vi "DAQ_software.vi"() -> ()   [LabVIEW 2014]
uses:
  <vilib>/Utility/file.llb/Write To Spreadsheet File (string).vi
panel:
  in  "recTime":dbl
  out "elapsed time":string
  out "end time":string
  out "start time":string
  out "Plot 6":waveform(dbl)(graph)={"t0"=timestamp(3541407835.153924 s since 1904-01-01), "dt"=0.001, "Y"=[-0.04272921159212641, -0.04272921159212641, -0.04305886997433487, -0.04305886997433487, -0.04305886997433487, -0.0433885283565454, -0.04305886997433487, -0.04305886997433487, -0.043718186738758026, -0.0433885283565454, -0.04305886997433487, -0.04239955320992001, -0.04239955320992001, -0.04239955320992001, -0.04305886997433487, -0.04272921159212641, -0.04239955320992001, -0.04272921159212641, -0.04206989482771564, -0.04272921159212641, -0.04272921159212641, -0.04272921159212641, -0.04272921159212641, -0.04272921159212641, -0.04272921159212641, -0.04239955320992001, -0.04272921159212641, -0.04272921159212641, -0.04272921159212641, -0.04272921159212641, -0.04305886997433487, -0.04305886997433487, -0.04305886997433487, -0.04272921159212641, -0.04272921159212641, -0.04305886997433487, -0.04272921159212641, -0.04305886997433487, -0.04272921159212641, -0.04239955320992001, -0.04272921159212641, -0.04305886997433487, -0.04272921159212641, -0.04272921159212641, -0.04305886997433487, -0.04305886997433487, -0.04272921159212641, -0.04206989482771564, -0.04272921159212641, -0.04305886997433487, -0.04272921159212641, -0.04239955320992001, -0.04239955320992001, -0.04272921159212641, -0.04272921159212641, -0.04239955320992001, -0.04239955320992001, -0.04272921159212641, -0.04239955320992001, -0.04272921159212641, -0.04239955320992001, -0.04272921159212641, -0.04239955320992001, -0.04239955320992001, -0.04239955320992001, -0.04305886997433487, -0.04305886997433487, -0.04305886997433487, -0.04305886997433487, -0.04272921159212641, -0.04305886997433487, -0.04272921159212641, -0.04239955320992001, -0.04239955320992001, -0.04305886997433487, -0.04239955320992001, -0.04239955320992001, -0.04239955320992001, -0.04239955320992001, -0.04272921159212641, -0.04272921159212641, -0.04239955320992001, -0.04239955320992001, -0.04239955320992001, -0.04239955320992001, -0.04239955320992001, -0.04239955320992001, -0.04272921159212641, -0.04272921159212641, -0.04305886997433487, -0.04272921159212641, -0.04272921159212641, -0.04272921159212641, -0.04272921159212641, -0.04272921159212641, -0.04272921159212641, -0.04239955320992001, -0.04239955320992001, -0.04272921159212641, -0.04272921159212641], "attributes"=variant("NI_ChannelName"=variant(string "ch1"), "NI_UnitDescription"=variant(string "Volts"))}
  out "Plot 5":waveform(dbl)(graph)={"t0"=timestamp(3541407835.153924 s since 1904-01-01), "dt"=0.001, "Y"=[-0.04272921159212641, -0.04272921159212641, -0.04305886997433487, -0.04305886997433487, -0.04305886997433487, -0.0433885283565454, -0.04305886997433487, -0.04305886997433487, -0.043718186738758026, -0.0433885283565454, -0.04305886997433487, -0.04239955320992001, -0.04239955320992001, -0.04239955320992001, -0.04305886997433487, -0.04272921159212641, -0.04239955320992001, -0.04272921159212641, -0.04206989482771564, -0.04272921159212641, -0.04272921159212641, -0.04272921159212641, -0.04272921159212641, -0.04272921159212641, -0.04272921159212641, -0.04239955320992001, -0.04272921159212641, -0.04272921159212641, -0.04272921159212641, -0.04272921159212641, -0.04305886997433487, -0.04305886997433487, -0.04305886997433487, -0.04272921159212641, -0.04272921159212641, -0.04305886997433487, -0.04272921159212641, -0.04305886997433487, -0.04272921159212641, -0.04239955320992001, -0.04272921159212641, -0.04305886997433487, -0.04272921159212641, -0.04272921159212641, -0.04305886997433487, -0.04305886997433487, -0.04272921159212641, -0.04206989482771564, -0.04272921159212641, -0.04305886997433487, -0.04272921159212641, -0.04239955320992001, -0.04239955320992001, -0.04272921159212641, -0.04272921159212641, -0.04239955320992001, -0.04239955320992001, -0.04272921159212641, -0.04239955320992001, -0.04272921159212641, -0.04239955320992001, -0.04272921159212641, -0.04239955320992001, -0.04239955320992001, -0.04239955320992001, -0.04305886997433487, -0.04305886997433487, -0.04305886997433487, -0.04305886997433487, -0.04272921159212641, -0.04305886997433487, -0.04272921159212641, -0.04239955320992001, -0.04239955320992001, -0.04305886997433487, -0.04239955320992001, -0.04239955320992001, -0.04239955320992001, -0.04239955320992001, -0.04272921159212641, -0.04272921159212641, -0.04239955320992001, -0.04239955320992001, -0.04239955320992001, -0.04239955320992001, -0.04239955320992001, -0.04239955320992001, -0.04272921159212641, -0.04272921159212641, -0.04305886997433487, -0.04272921159212641, -0.04272921159212641, -0.04272921159212641, -0.04272921159212641, -0.04272921159212641, -0.04272921159212641, -0.04239955320992001, -0.04239955320992001, -0.04272921159212641, -0.04272921159212641], "attributes"=variant("NI_ChannelName"=variant(string "ch1"), "NI_UnitDescription"=variant(string "Volts"))}
  out "Plot 4":waveform(dbl)(graph)={"t0"=timestamp(3541407835.153924 s since 1904-01-01), "dt"=0.001, "Y"=[-0.04272921159212641, -0.04272921159212641, -0.04305886997433487, -0.04305886997433487, -0.04305886997433487, -0.0433885283565454, -0.04305886997433487, -0.04305886997433487, -0.043718186738758026, -0.0433885283565454, -0.04305886997433487, -0.04239955320992001, -0.04239955320992001, -0.04239955320992001, -0.04305886997433487, -0.04272921159212641, -0.04239955320992001, -0.04272921159212641, -0.04206989482771564, -0.04272921159212641, -0.04272921159212641, -0.04272921159212641, -0.04272921159212641, -0.04272921159212641, -0.04272921159212641, -0.04239955320992001, -0.04272921159212641, -0.04272921159212641, -0.04272921159212641, -0.04272921159212641, -0.04305886997433487, -0.04305886997433487, -0.04305886997433487, -0.04272921159212641, -0.04272921159212641, -0.04305886997433487, -0.04272921159212641, -0.04305886997433487, -0.04272921159212641, -0.04239955320992001, -0.04272921159212641, -0.04305886997433487, -0.04272921159212641, -0.04272921159212641, -0.04305886997433487, -0.04305886997433487, -0.04272921159212641, -0.04206989482771564, -0.04272921159212641, -0.04305886997433487, -0.04272921159212641, -0.04239955320992001, -0.04239955320992001, -0.04272921159212641, -0.04272921159212641, -0.04239955320992001, -0.04239955320992001, -0.04272921159212641, -0.04239955320992001, -0.04272921159212641, -0.04239955320992001, -0.04272921159212641, -0.04239955320992001, -0.04239955320992001, -0.04239955320992001, -0.04305886997433487, -0.04305886997433487, -0.04305886997433487, -0.04305886997433487, -0.04272921159212641, -0.04305886997433487, -0.04272921159212641, -0.04239955320992001, -0.04239955320992001, -0.04305886997433487, -0.04239955320992001, -0.04239955320992001, -0.04239955320992001, -0.04239955320992001, -0.04272921159212641, -0.04272921159212641, -0.04239955320992001, -0.04239955320992001, -0.04239955320992001, -0.04239955320992001, -0.04239955320992001, -0.04239955320992001, -0.04272921159212641, -0.04272921159212641, -0.04305886997433487, -0.04272921159212641, -0.04272921159212641, -0.04272921159212641, -0.04272921159212641, -0.04272921159212641, -0.04272921159212641, -0.04239955320992001, -0.04239955320992001, -0.04272921159212641, -0.04272921159212641], "attributes"=variant("NI_ChannelName"=variant(string "ch1"), "NI_UnitDescription"=variant(string "Volts"))}
  out "Plot 3":waveform(dbl)(graph)={"t0"=timestamp(3541407835.153924 s since 1904-01-01), "dt"=0.001, "Y"=[-0.04272921159212641, -0.04272921159212641, -0.04305886997433487, -0.04305886997433487, -0.04305886997433487, -0.0433885283565454, -0.04305886997433487, -0.04305886997433487, -0.043718186738758026, -0.0433885283565454, -0.04305886997433487, -0.04239955320992001, -0.04239955320992001, -0.04239955320992001, -0.04305886997433487, -0.04272921159212641, -0.04239955320992001, -0.04272921159212641, -0.04206989482771564, -0.04272921159212641, -0.04272921159212641, -0.04272921159212641, -0.04272921159212641, -0.04272921159212641, -0.04272921159212641, -0.04239955320992001, -0.04272921159212641, -0.04272921159212641, -0.04272921159212641, -0.04272921159212641, -0.04305886997433487, -0.04305886997433487, -0.04305886997433487, -0.04272921159212641, -0.04272921159212641, -0.04305886997433487, -0.04272921159212641, -0.04305886997433487, -0.04272921159212641, -0.04239955320992001, -0.04272921159212641, -0.04305886997433487, -0.04272921159212641, -0.04272921159212641, -0.04305886997433487, -0.04305886997433487, -0.04272921159212641, -0.04206989482771564, -0.04272921159212641, -0.04305886997433487, -0.04272921159212641, -0.04239955320992001, -0.04239955320992001, -0.04272921159212641, -0.04272921159212641, -0.04239955320992001, -0.04239955320992001, -0.04272921159212641, -0.04239955320992001, -0.04272921159212641, -0.04239955320992001, -0.04272921159212641, -0.04239955320992001, -0.04239955320992001, -0.04239955320992001, -0.04305886997433487, -0.04305886997433487, -0.04305886997433487, -0.04305886997433487, -0.04272921159212641, -0.04305886997433487, -0.04272921159212641, -0.04239955320992001, -0.04239955320992001, -0.04305886997433487, -0.04239955320992001, -0.04239955320992001, -0.04239955320992001, -0.04239955320992001, -0.04272921159212641, -0.04272921159212641, -0.04239955320992001, -0.04239955320992001, -0.04239955320992001, -0.04239955320992001, -0.04239955320992001, -0.04239955320992001, -0.04272921159212641, -0.04272921159212641, -0.04305886997433487, -0.04272921159212641, -0.04272921159212641, -0.04272921159212641, -0.04272921159212641, -0.04272921159212641, -0.04272921159212641, -0.04239955320992001, -0.04239955320992001, -0.04272921159212641, -0.04272921159212641], "attributes"=variant("NI_ChannelName"=variant(string "ch1"), "NI_UnitDescription"=variant(string "Volts"))}
  out "Plot 2":waveform(dbl)(graph)={"t0"=timestamp(3541407835.153924 s since 1904-01-01), "dt"=0.001, "Y"=[-0.04272921159212641, -0.04272921159212641, -0.04305886997433487, -0.04305886997433487, -0.04305886997433487, -0.0433885283565454, -0.04305886997433487, -0.04305886997433487, -0.043718186738758026, -0.0433885283565454, -0.04305886997433487, -0.04239955320992001, -0.04239955320992001, -0.04239955320992001, -0.04305886997433487, -0.04272921159212641, -0.04239955320992001, -0.04272921159212641, -0.04206989482771564, -0.04272921159212641, -0.04272921159212641, -0.04272921159212641, -0.04272921159212641, -0.04272921159212641, -0.04272921159212641, -0.04239955320992001, -0.04272921159212641, -0.04272921159212641, -0.04272921159212641, -0.04272921159212641, -0.04305886997433487, -0.04305886997433487, -0.04305886997433487, -0.04272921159212641, -0.04272921159212641, -0.04305886997433487, -0.04272921159212641, -0.04305886997433487, -0.04272921159212641, -0.04239955320992001, -0.04272921159212641, -0.04305886997433487, -0.04272921159212641, -0.04272921159212641, -0.04305886997433487, -0.04305886997433487, -0.04272921159212641, -0.04206989482771564, -0.04272921159212641, -0.04305886997433487, -0.04272921159212641, -0.04239955320992001, -0.04239955320992001, -0.04272921159212641, -0.04272921159212641, -0.04239955320992001, -0.04239955320992001, -0.04272921159212641, -0.04239955320992001, -0.04272921159212641, -0.04239955320992001, -0.04272921159212641, -0.04239955320992001, -0.04239955320992001, -0.04239955320992001, -0.04305886997433487, -0.04305886997433487, -0.04305886997433487, -0.04305886997433487, -0.04272921159212641, -0.04305886997433487, -0.04272921159212641, -0.04239955320992001, -0.04239955320992001, -0.04305886997433487, -0.04239955320992001, -0.04239955320992001, -0.04239955320992001, -0.04239955320992001, -0.04272921159212641, -0.04272921159212641, -0.04239955320992001, -0.04239955320992001, -0.04239955320992001, -0.04239955320992001, -0.04239955320992001, -0.04239955320992001, -0.04272921159212641, -0.04272921159212641, -0.04305886997433487, -0.04272921159212641, -0.04272921159212641, -0.04272921159212641, -0.04272921159212641, -0.04272921159212641, -0.04272921159212641, -0.04239955320992001, -0.04239955320992001, -0.04272921159212641, -0.04272921159212641], "attributes"=variant("NI_ChannelName"=variant(string "ch1"), "NI_UnitDescription"=variant(string "Volts"))}
  in  "dm6":dbl=1.0
  in  "do6":dbl
  in  "dm5":dbl=1.0
  in  "do5":dbl
  in  "dm4":dbl=1.0
  in  "do4":dbl
  in  "dm3":dbl=1.0
  in  "do3":dbl
  in  "dm2":dbl=1.0
  in  "do2":dbl
  in  "do1":dbl
  in  "dm1":dbl=1.0
  out "Plot 1":waveform(dbl)(graph)={"t0"=timestamp(3541407835.153924 s since 1904-01-01), "dt"=0.001, "Y"=[-0.04272921159212641, -0.04272921159212641, -0.04305886997433487, -0.04305886997433487, -0.04305886997433487, -0.0433885283565454, -0.04305886997433487, -0.04305886997433487, -0.043718186738758026, -0.0433885283565454, -0.04305886997433487, -0.04239955320992001, -0.04239955320992001, -0.04239955320992001, -0.04305886997433487, -0.04272921159212641, -0.04239955320992001, -0.04272921159212641, -0.04206989482771564, -0.04272921159212641, -0.04272921159212641, -0.04272921159212641, -0.04272921159212641, -0.04272921159212641, -0.04272921159212641, -0.04239955320992001, -0.04272921159212641, -0.04272921159212641, -0.04272921159212641, -0.04272921159212641, -0.04305886997433487, -0.04305886997433487, -0.04305886997433487, -0.04272921159212641, -0.04272921159212641, -0.04305886997433487, -0.04272921159212641, -0.04305886997433487, -0.04272921159212641, -0.04239955320992001, -0.04272921159212641, -0.04305886997433487, -0.04272921159212641, -0.04272921159212641, -0.04305886997433487, -0.04305886997433487, -0.04272921159212641, -0.04206989482771564, -0.04272921159212641, -0.04305886997433487, -0.04272921159212641, -0.04239955320992001, -0.04239955320992001, -0.04272921159212641, -0.04272921159212641, -0.04239955320992001, -0.04239955320992001, -0.04272921159212641, -0.04239955320992001, -0.04272921159212641, -0.04239955320992001, -0.04272921159212641, -0.04239955320992001, -0.04239955320992001, -0.04239955320992001, -0.04305886997433487, -0.04305886997433487, -0.04305886997433487, -0.04305886997433487, -0.04272921159212641, -0.04305886997433487, -0.04272921159212641, -0.04239955320992001, -0.04239955320992001, -0.04305886997433487, -0.04239955320992001, -0.04239955320992001, -0.04239955320992001, -0.04239955320992001, -0.04272921159212641, -0.04272921159212641, -0.04239955320992001, -0.04239955320992001, -0.04239955320992001, -0.04239955320992001, -0.04239955320992001, -0.04239955320992001, -0.04272921159212641, -0.04272921159212641, -0.04305886997433487, -0.04272921159212641, -0.04272921159212641, -0.04272921159212641, -0.04272921159212641, -0.04272921159212641, -0.04272921159212641, -0.04239955320992001, -0.04239955320992001, -0.04272921159212641, -0.04272921159212641], "attributes"=variant("NI_ChannelName"=variant(string "ch1"), "NI_UnitDescription"=variant(string "Volts"))}
  in  "chNames":string[](array[string])=["Channel 1", "Channel 2", "Channel 3"]
  in  "MeasInfo":string[][](table)=[["measurment name", "Energy Harvesting"], ["operator name", "Adrian Zurbuchen"], ["date", "21.03.16"]]
  in  "stop":bool
  in  "file name":string="experiment1_meas1"
  in  "file path":path=path "D:/Adrian/EnergyHarvesting/turbine eh"
  in  "record":bool
  out "rate":dbl=1000.0
  out "number of samples":i32=100
  # "display multiplier:"
  # "display offset:"
  # "display multiplier:"
  # "display offset:"
  # "data acquisition settings"
  # "Start/Stop Recording"
  # "display multiplier:"
  # "display offset:"
  # "display multiplier:"
  # "display offset:"
  # "s"
  # "rec time (0: disabled)"
  # "Measurment Info"
  # "display multiplier:"
  # "display offset:"
  # "display multiplier:"
  # "display offset:"
  # "Channel Names"
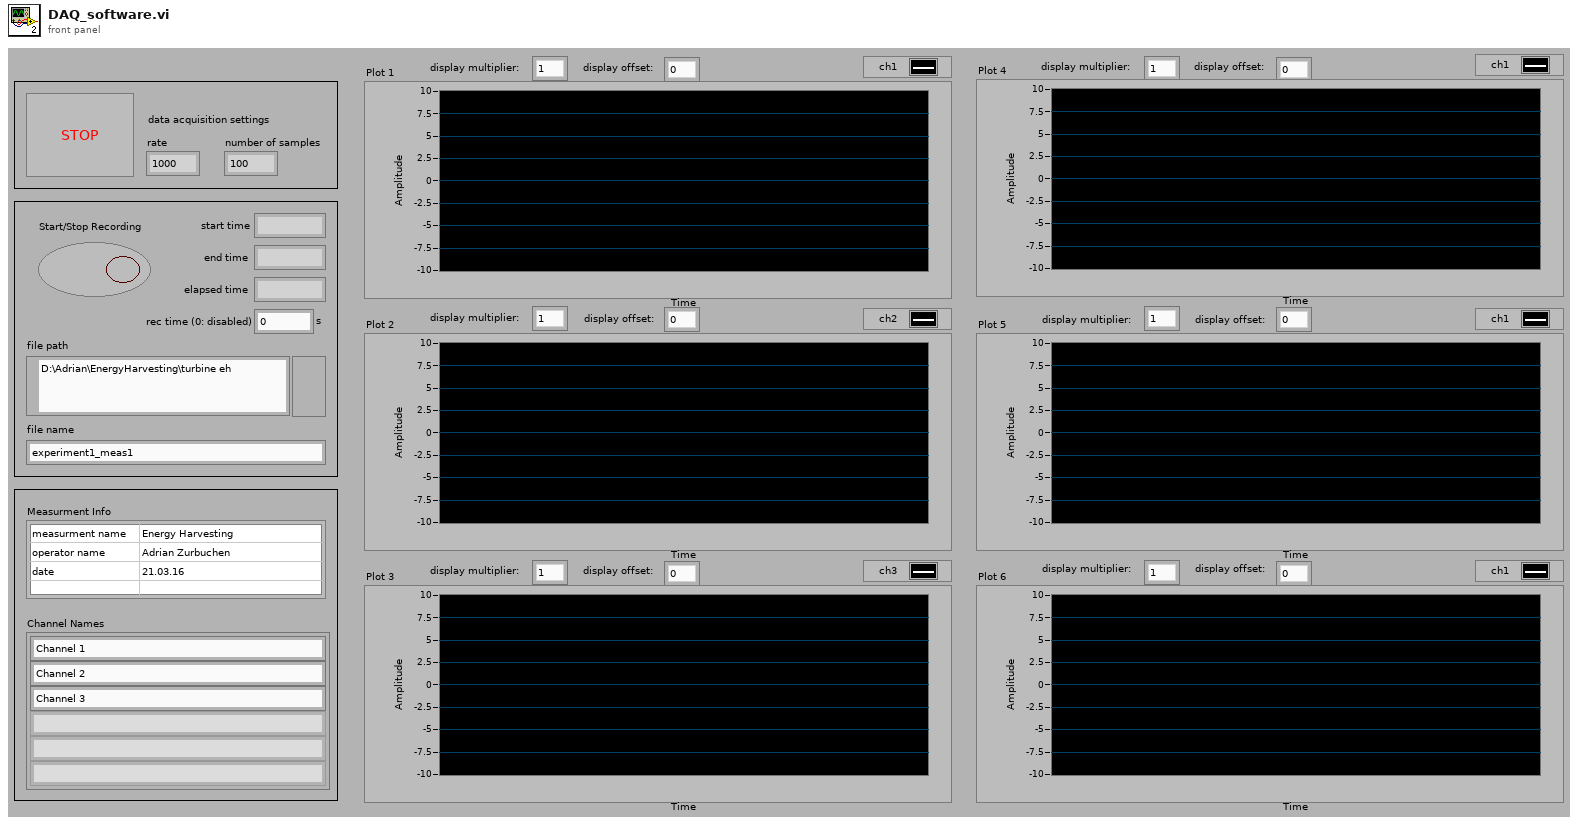
[diagram p1: front panel]
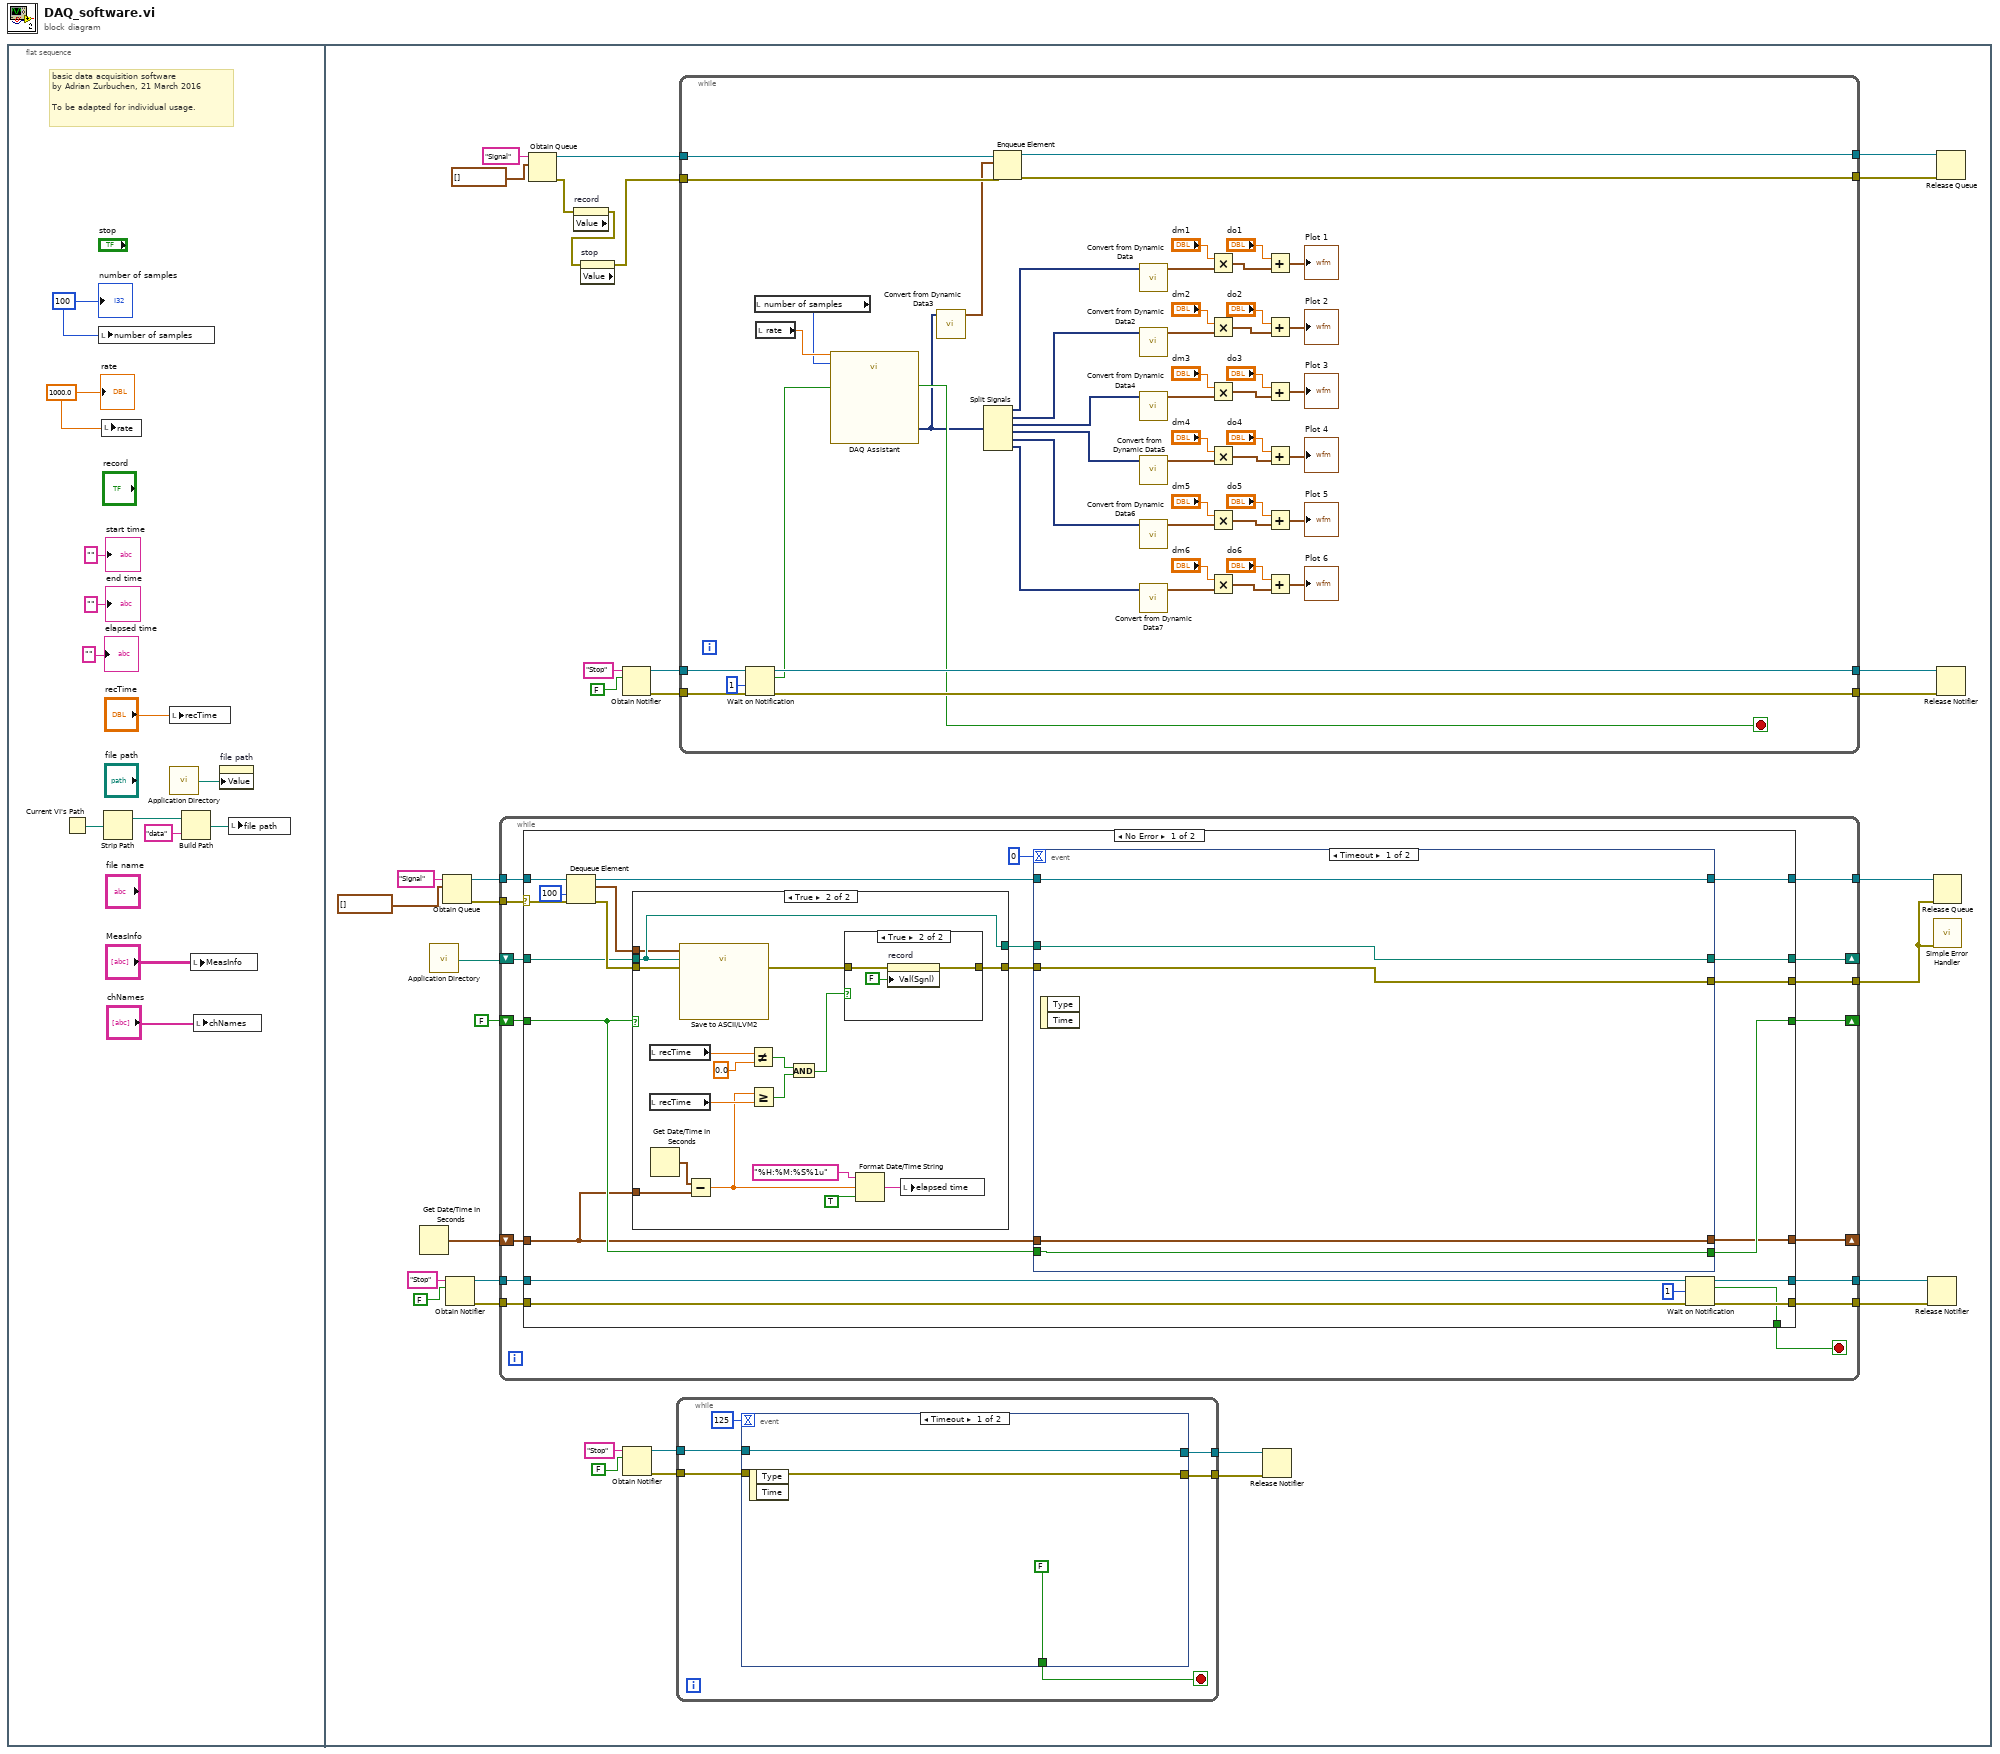
[diagram p0: block diagram]
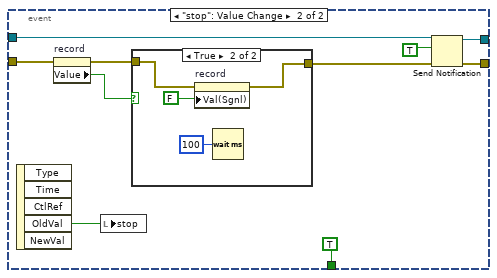
[diagram p2: hidden frame]
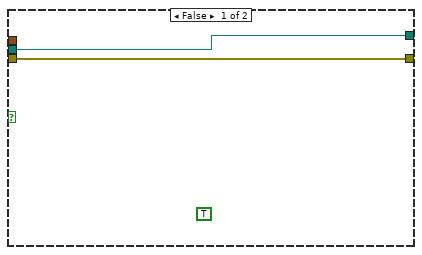
[diagram p4: hidden frame]
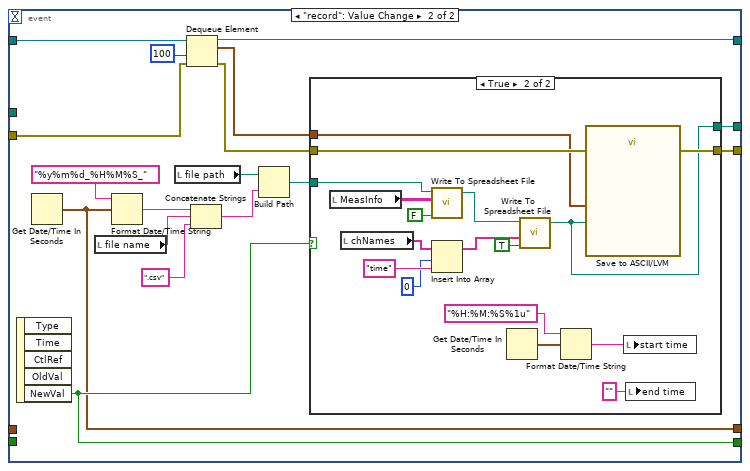
[diagram p6: hidden frame]
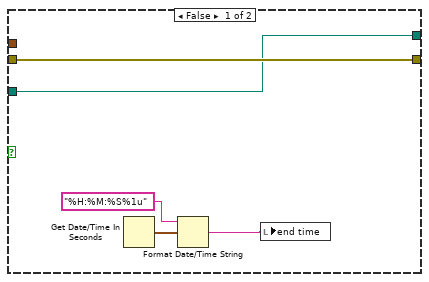
[diagram p7: hidden frame]
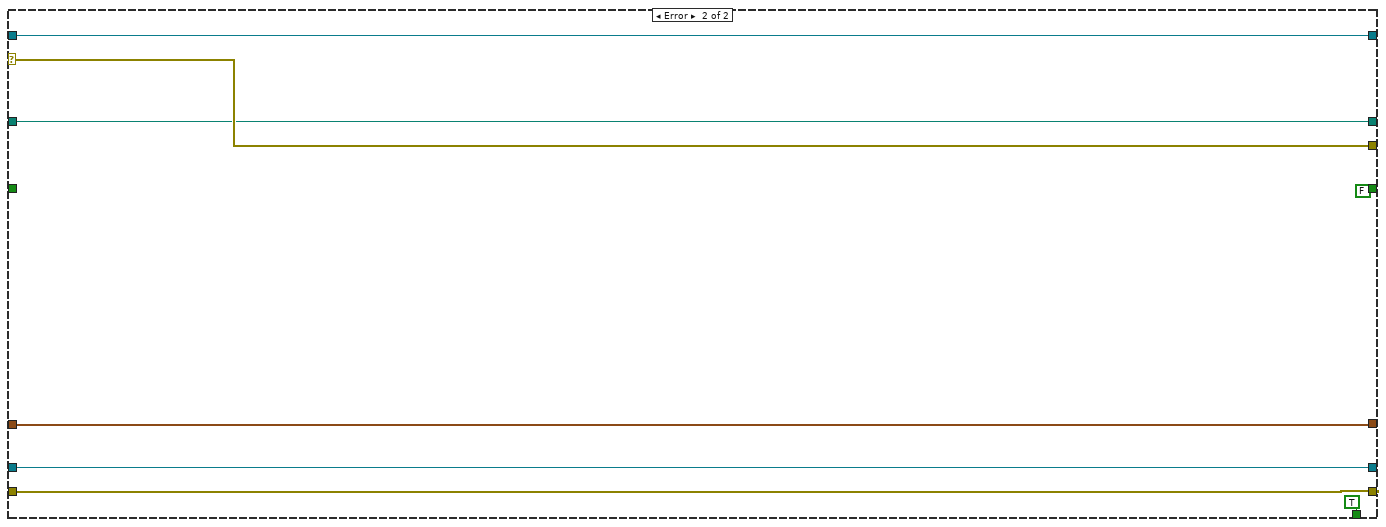
[diagram p8: hidden frame]
diagram:
  n1 = flat-sequence {
    frame #0 {
      w12 = 100 ("number of samples")
      w13 = 1000.0 ("rate")
      # "basic data acquisition software\nby Adrian Zurbuchen, 21 March 2016\n\nTo be adapted for individual usage."
      n2 = Current VI's Path() -> (path=w9:path)
      n3 = local write "number of samples"(w12) -> ()
      n4 = local write "rate"(w13) -> ()
      n5 = Strip Path(path=w9) -> (stripped path=w8:path)  [unwired: 1 out]
      n6 = local write "recTime"("recTime") -> ()
      n7 = call <vilib>:"Application Directory.vi"() -> ("Application Directory"=w5:path)
      n8 = Build Path(base path=w8, name or relative path="data") -> (appended path=w10:path)
      n9 = local write "MeasInfo"("MeasInfo") -> ()
      n10 = local write "chNames"("chNames") -> ()
      n11 = property on="file path" class="Path"("Value"=w5) -> ()  [unwired: 2 in, 2 out]
      n12 = local write "file path"(w10) -> ()
      "number of samples" <- w12
      "rate" <- w13
      "elapsed time" <- "" ("elapsed time")
      "end time" <- "" ("end time")
      "start time" <- "" ("start time")
    }
    frame #1 {
      n13 = Get Date/Time In Seconds() -> (seconds since 1Jan1904=w14:timestamp)
      n14 = call <vilib>:"Application Directory.vi"() -> ("Application Directory"=w15:path)
      n15 = Obtain Queue(name (unnamed)="Signal", element data type=waveform(dbl)[] [] ("Array of Waveform")) -> (queue out=w42:refnum<queue>, error out=w41:errorcluster)  [unwired: 3 in, 1 out]
      n16 = Obtain Notifier(name (unnamed)="Stop", notification data type=FALSE ("NewVal")) -> (notifier out=w26:refnum<notifier>, error out=w25:errorcluster)  [unwired: 2 in, 1 out]
      n17 = while {
        tunnel: w42 -> [w85]
        tunnel: w41 -> [w87]
        shift-right: [w83] -> _
        shift-left: FALSE ("NewVal") -> [w84]
        tunnel: [w82] -> w40
        tunnel: [w81] -> w18
        tunnel: [w80] -> w28
        tunnel: [w79] -> w27
        tunnel: w26 -> [w78]
        tunnel: w25 -> [w77]
        shift-right: [w76] -> _
        shift-left: w15 -> [w75]
        shift-right: [w74] -> _
        shift-left: w14 -> [w73]
        stop <- w86 stop-if-true
        n18 = case shown="No Error" w87 {
          selector: w87 -> [w109 w183]
          tunnel: [w95 TRUE] -> w86
          tunnel: w85 -> [w110 w182]
          tunnel: [w90 w182] -> w82
          tunnel: [w96 FALSE ("NewVal")] -> w83
          tunnel: w84 -> [w106 _]
          tunnel: [w104 w183] -> w81
          tunnel: [w101 w181] -> w80
          tunnel: [w100 w180] -> w79
          tunnel: w78 -> [w99 w181]
          tunnel: w77 -> [w98 w180]
          tunnel: [w94 w179] -> w76
          tunnel: w75 -> [w93 w179]
          tunnel: [w89 w178] -> w74
          tunnel: w73 -> [w88 w178]
          frame No Error {
            n19 = Dequeue Element(queue=w110, timeout in ms (-1)=100, error in (no error)=w109) -> (queue out=w91:refnum<queue>, element=w103:waveform(dbl)[], error out=w108:errorcluster)  [unwired: 1 out]
            n20 = case shown="True" w106 {
              tunnel: w108 -> [w112 w128]
              tunnel: [w112 w120] -> w105
              tunnel: w103 -> [_ w127]
              tunnel: w93 -> [w111 w129]
              tunnel: [w111 w129] -> w92
              tunnel: w88 -> [_ w125]
              frame False {
                (unwired) TRUE ("Reset")
              }
              frame True {
                n21 = local read "recTime"() -> (w115:dbl)
                n22 = local read "recTime"() -> (w119:dbl)
                n23 = Get Date/Time In Seconds() -> (seconds since 1Jan1904=w126:timestamp)
                n24 = call "Save to ASCII/LVM2"("signals in"=w127, "File Path"=w129, "error in"=w128) -> ("error out"=w121:errorcluster)  [unwired: 16 in]
                n25 = Subtract(x=w126, y=w125) -> (x-y=w113:dbl)
                n26 = Not Equal?(x=w115, y=0.0) -> (x != y?=w116:bool)
                n27 = Greater Or Equal?(x=w113, y=w119) -> (x >= y?=w118:bool)
                n28 = And(x=w116, y=w118) -> (x .and. y?=w117:bool)
                n29 = case shown="True" w117 {
                  tunnel: w121 -> [w130 w132]
                  tunnel: [w130 w131] -> w120
                  frame False {
                  }
                  frame True {
                    n30 = property on="record" class="Bool (strict)"(error in=w132, "Val(Sgnl)"=FALSE ("Value (Signaling)")) -> (error out=w131:errorcluster)  [unwired: 1 in, 1 out]
                  }
                }
                n31 = Format Date/Time String(time format string (%c)="%H:%M:%S%1u", seconds (now)=w113, UTC format=TRUE) -> (date/time string=w123:string)
                n32 = local write "elapsed time"(w123) -> ()
              }
            }
            n33 = event shown="[0] Timeout" {
              selector: _ -> [_ _]
              dyn-events: _ -> [_ _]
              timeout: 0 -> [_ _]
              tunnel: [w138 w149] -> w96
              tunnel: w106 -> [w138 _]
              tunnel: w105 -> [w137 w142]
              tunnel: [w137 w148] -> w104
              tunnel: [w136 w146] -> w94
              tunnel: w92 -> [w136 _]
              tunnel: w91 -> [w135 w145]
              tunnel: [w135 w144] -> w90
              tunnel: [w134 w139] -> w89
              tunnel: w88 -> [w134 _]
              event Timeout {
                n34 = event-data() -> ()  [unwired: 1 in, 2 out]
              }
              event "record": Value Change {
                n35 = event-data() -> ("NewVal"=w149:bool)  [unwired: 1 in, 4 out]
                n36 = Get Date/Time In Seconds() -> (seconds since 1Jan1904=w139:timestamp)
                n37 = local read "file name"() -> (w152:string)
                n38 = Format Date/Time String(time format string (%c)="%y%m%d_%H%M%S_", seconds (now)=w139) -> (date/time string=w154:string)  [unwired: 1 in]
                n39 = local read "file path"() -> (w151:path)
                n40 = Dequeue Element(queue=w145, timeout in ms (-1)=100, error in (no error)=w142) -> (queue out=w144:refnum<queue>, element=w140:waveform(dbl)[], error out=w141:errorcluster)  [unwired: 1 out]
                n41 = Concatenate Strings(w154, w152, ".csv" ("string")) -> (w150:string)
                n42 = Build Path(base path=w151, name or relative path=w150) -> (appended path=w147:path)
                n43 = case shown="True" w149 {
                  tunnel: [w160 w176] -> w148
                  tunnel: w147 -> [w159 w173]
                  tunnel: w141 -> [w160 w177]
                  tunnel: [w159 w169] -> w146
                  tunnel: w140 -> [_ w175]
                  frame False {
                    n44 = Get Date/Time In Seconds() -> (seconds since 1Jan1904=w158:timestamp)
                    n45 = Format Date/Time String(time format string (%c)="%H:%M:%S%1u", seconds (now)=w158) -> (date/time string=w156:string)  [unwired: 1 in]
                    n46 = local write "end time"(w156) -> ()
                  }
                  frame True {
                    n47 = local read "MeasInfo"() -> (w174:string[][])
                    n48 = local read "chNames"() -> (w167:string[])
                    n49 = call-poly <vilib>:"Write To Spreadsheet File.vi"("append to file? (new file:F)"=FALSE, "2D data"=w174, "file path (dialog if empty)"=w173) -> ("new file path (Not A Path if cancelled)"=w171:path)  [unwired: 5 in]
                    n50 = Insert Into Array(array=w167, index=0, new element="time") -> (w165:string[])
                    n51 = Get Date/Time In Seconds() -> (seconds since 1Jan1904=w164:timestamp)
                    n52 = call-poly <vilib>:"Write To Spreadsheet File.vi"("append to file? (new file:F)"=TRUE, "1D data"=w165, "file path (dialog if empty)"=w171) -> ("new file path (Not A Path if cancelled)"=w169:path)  [unwired: 5 in]
                    n53 = Format Date/Time String(time format string (%c)="%H:%M:%S%1u", seconds (now)=w164) -> (date/time string=w162:string)  [unwired: 1 in]
                    n54 = call "Save to ASCII/LVM"("signals in"=w175, "File Path"=w169, "error in"=w177) -> ("error out"=w176:errorcluster)  [unwired: 16 in]
                    n55 = local write "start time"(w162) -> ()
                    n56 = local write "end time"("" ("end time")) -> ()
                  }
                }
              }
            }
            n57 = Wait on Notification(notifier=w99, timeout in ms (-1)=1, error in (no error)=w98) -> (notifier out=w101:refnum<notifier>, notification=w95:bool, error out=w100:errorcluster)  [unwired: 1 in, 1 out]
          }
          frame Error {
          }
        }
      }
      n58 = Obtain Queue(name (unnamed)="Signal", element data type=waveform(dbl)[] [] ("Array of Waveform")) -> (queue out=w47:refnum<queue>, error out=w44:errorcluster)  [unwired: 3 in, 1 out]
      n59 = property on="record" class="Bool (strict)" props=["Value"](error in=w44) -> (error out=w38:errorcluster)  [unwired: 1 in, 2 out]
      n60 = property on="stop" class="Bool (strict)" props=["Value"](error in=w38) -> (error out=w37:errorcluster)  [unwired: 1 in, 2 out]
      n61 = Obtain Notifier(name (unnamed)="Stop", notification data type=FALSE ("NewVal")) -> (notifier out=w34:refnum<notifier>, error out=w33:errorcluster)  [unwired: 2 in, 1 out]
      n62 = Obtain Notifier(name (unnamed)="Stop", notification data type=FALSE ("NewVal")) -> (notifier out=w22:refnum<notifier>, error out=w21:errorcluster)  [unwired: 2 in, 1 out]
      n63 = while {
        tunnel: w22 -> [w54]
        tunnel: w21 -> [w53]
        tunnel: [w52] -> w19
        tunnel: [w51] -> w20
        stop <- w50 stop-if-true
        n64 = event shown="[0] Timeout" {
          selector: _ -> [_ _]
          dyn-events: _ -> [_ _]
          timeout: 125 -> [_ _]
          tunnel: w54 -> [w57 w63]
          tunnel: w53 -> [w56 w59]
          tunnel: [w56 w64] -> w52
          tunnel: [w57 w65] -> w51
          tunnel: [FALSE ("notification") TRUE ("notification")] -> w50
          event Timeout {
            n65 = event-data() -> ()  [unwired: 1 in, 2 out]
          }
          event "stop": Value Change {
            n66 = event-data() -> ("OldVal"=w67:bool)  [unwired: 1 in, 4 out]
            n67 = property on="record" class="Bool (strict)"(error in=w59) -> (error out=w58:errorcluster, "Value"=w60:bool)  [unwired: 1 in, 1 out]
            n68 = local write "stop"(w67) -> ()
            n69 = case shown="True" w60 {
              tunnel: w58 -> [w68 w69]
              tunnel: [w68 w71] -> w61
              frame False {
              }
              frame True {
                n70 = property on="record" class="Bool (strict)"(error in=w69, "Val(Sgnl)"=FALSE ("Record")) -> (error out=w71:errorcluster)  [unwired: 1 in, 1 out]
                n71 = Wait (ms)(milliseconds to wait=u32 100) -> ()  [unwired: 1 out]
              }
            }
            n72 = Send Notification(notification=TRUE, notifier=w63, error in (no error)=w61) -> (notifier out=w65:refnum<notifier>, error out=w64:errorcluster)
          }
        }
      }
      n73 = while {
        tunnel: w47 -> [w236]
        tunnel: w37 -> [w235]
        tunnel: [w234] -> w46
        tunnel: [w216] -> w45
        tunnel: w34 -> [w232]
        tunnel: w33 -> [w231]
        tunnel: [w233] -> w32
        tunnel: [w229] -> w31
        stop <- w227 stop-if-true
        n74 = Wait on Notification(notifier=w232, timeout in ms (-1)=1, error in (no error)=w231) -> (notifier out=w233:refnum<notifier>, notification=w228:bool, error out=w229:errorcluster)  [unwired: 1 in, 1 out]
        n75 = local read "number of samples"() -> (w225:i32)
        n76 = local read "rate"() -> (w226:dbl)
        n77 = call "DAQ Assistant"("rate"=w226, "number of samples"=w225, "stop (F)"=w228) -> ("data"=w223:dynamicdata, "stopped"=w227:bool)  [unwired: 13 in, 2 out]
        n78 = call "Convert from Dynamic Data3"("Dynamic Data Type"=w223) -> ("Array of Waveform"=w224:waveform(dbl)[])  [unwired: 3 in]
        n79 = Split Signals(w223) -> (w222:dynamicdata, w221:dynamicdata, w220:dynamicdata, w219:dynamicdata, w218:dynamicdata, w217:dynamicdata)  [unwired: 6 in]
        n80 = Enqueue Element(queue=w236, element=w224, error in (no error)=w235) -> (queue out=w234:refnum<queue>, error out=w216:errorcluster)  [unwired: 1 in, 1 out]
        n81 = call "Convert from Dynamic Data"("Dynamic Data Type"=w222) -> ("Waveform"=w214:waveform(dbl))  [unwired: 3 in]
        n82 = call "Convert from Dynamic Data2"("Dynamic Data Type"=w221) -> ("Waveform"=w207:waveform(dbl))  [unwired: 3 in]
        n83 = call "Convert from Dynamic Data4"("Dynamic Data Type"=w220) -> ("Waveform"=w194:waveform(dbl))  [unwired: 3 in]
        n84 = call "Convert from Dynamic Data5"("Dynamic Data Type"=w219) -> ("Waveform"=w193:waveform(dbl))  [unwired: 3 in]
        n85 = call "Convert from Dynamic Data6"("Dynamic Data Type"=w218) -> ("Waveform"=w192:waveform(dbl))  [unwired: 3 in]
        n86 = call "Convert from Dynamic Data7"("Dynamic Data Type"=w217) -> ("Waveform"=w191:waveform(dbl))  [unwired: 3 in]
        n87 = Multiply(x="dm1", y=w214) -> (x*y=w213:waveform(dbl))
        n88 = Multiply(x="dm2", y=w207) -> (x*y=w209:waveform(dbl))
        n89 = Multiply(x="dm3", y=w194) -> (x*y=w205:waveform(dbl))
        n90 = Multiply(x="dm4", y=w193) -> (x*y=w202:waveform(dbl))
        n91 = Multiply(x="dm5", y=w192) -> (x*y=w199:waveform(dbl))
        n92 = Multiply(x="dm6", y=w191) -> (x*y=w196:waveform(dbl))
        n93 = Add(x="do1", y=w213) -> (x+y=→"Plot 1":waveform(dbl))
        n94 = Add(x="do2", y=w209) -> (x+y=→"Plot 2":waveform(dbl))
        n95 = Add(x="do3", y=w205) -> (x+y=→"Plot 3":waveform(dbl))
        n96 = Add(x="do4", y=w202) -> (x+y=→"Plot 4":waveform(dbl))
        n97 = Add(x="do5", y=w199) -> (x+y=→"Plot 5":waveform(dbl))
        n98 = Add(x="do6", y=w196) -> (x+y=→"Plot 6":waveform(dbl))
      }
      n99 = Release Notifier(notifier=w20, error in (no error)=w19) -> ()  [unwired: 1 in, 3 out]
      n100 = Release Notifier(notifier=w28, error in (no error)=w27) -> ()  [unwired: 1 in, 3 out]
      n101 = Release Queue(queue=w40, error in (no error)=w18) -> ()  [unwired: 1 in, 3 out]
      n102 = call <vilib>:"Simple Error Handler.vi"("error in (no error)"=w18) -> ()  [unwired: 4 in, 5 out]
      n103 = Release Queue(queue=w46, error in (no error)=w45) -> ()  [unwired: 1 in, 3 out]
      n104 = Release Notifier(notifier=w32, error in (no error)=w31) -> ()  [unwired: 1 in, 3 out]
    }
  }
